vi "Download.vi"(5 "ICommunicate":refnum<class "ICommunicate.lvclass">, 7 "Node-ID":u8, 8 "error in":errorcluster, 9 "Value":variant, 10 "Multiplexer":cluster{"Index":u16, "Sub-Index":u8} {"Index" format="%.0x"}, 11 "SDO Manager in":refnum<class "SDO Manager.lvclass">) -> (0 "error out":errorcluster, 2 "Success?":bool, 3 "SDO Manager out":refnum<class "SDO Manager.lvclass">)   [LabVIEW 2024, in "CANopen Master.lvlib" / "SDO Manager.lvclass"]
uses:
  SDO Manager.lvclass
  SDO Manager.lvclass/SDO Manager.ctl
  CANopen Request/CANopen Request Message.lvclass
  Service Data Object/Service Data Object.lvclass
  CANopen Message/CANopen Message.lvclass
  HAL/Source/Interfaces/ICommunicate/ICommunicate.lvclass
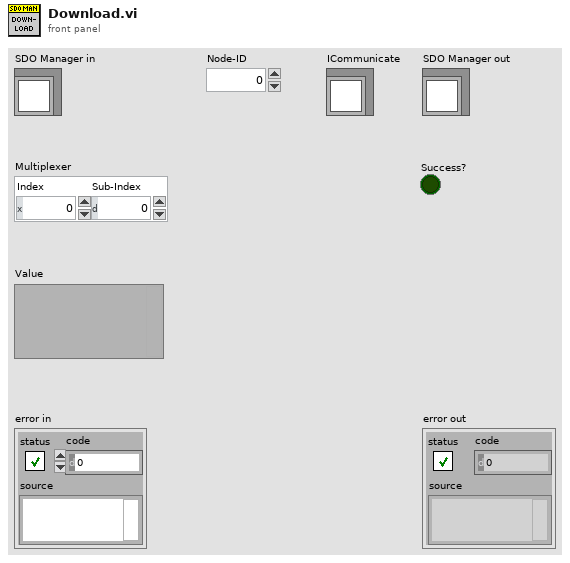
[diagram p1: front panel]
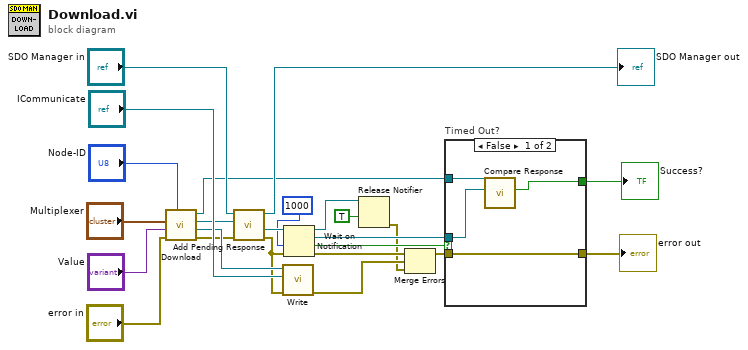
[diagram p0: block diagram]
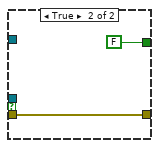
[diagram p2: hidden frame]
diagram:
  n1 = call "Download.vi"("Node-ID"="Node-ID", "error in"="error in", "Value"="Value", "Multiplexer"="Multiplexer") -> ("error out"=w7:errorcluster, "Request"=w17:refnum<class "CANopen Request Message.lvclass">, "Expected Response"=w16:refnum<class "CANopen Response Message.lvclass">, "Service Data Object out"=w12:refnum<class "Service Data Object.lvclass">)  [unwired: 4 in]
  n2 = call "Add Pending Response.vi"("Error In"=w7, "Expected Response"=w16, "reference in"="SDO Manager in") -> ("Error Out"=w3:errorcluster, "Response Notifier out"=w13:refnum<notifier>, "reference out"=→"SDO Manager out":refnum<class "SDO Manager.lvclass">)  [unwired: 6 in]
  n3 = call "Write.vi"("error in"=w3, "ICommunicate"="ICommunicate", "CANopen Message in"=w17) -> ("error out"=w2:errorcluster)  [unwired: 7 in, 1 out]
  n4 = Wait on Notification(notifier=w13, timeout in ms (-1)=1000, error in (no error)=w3) -> (notifier out=w6:refnum<notifier>, notification=w9:refnum<class "CANopen Response Message.lvclass">, timed out?=w8:bool, error out=w10:errorcluster)  [unwired: 1 in]
  n5 = Release Notifier(notifier=w6, force destroy? (F)=TRUE) -> (error out=w1:errorcluster)  [unwired: 1 in, 2 out]
  n6 = Merge Errors(w10, w2, w1) -> (w4:errorcluster)
  n7 = case "Timed Out?" shown="False" w8 {
    tunnel: w4 -> [w25 w30]
    tunnel: [w25 w30] -> w20
    tunnel: w9 -> [w27 _]
    tunnel: [w26 FALSE ("Equal?")] -> w19
    tunnel: w12 -> [w28 _]
    frame False {
      n8 = call "Compare Response.vi"("Actual"=w27, "Service Data Object"=w28) -> ("Equal?"=w26:bool)  [unwired: 8 in, 1 out]
    }
    frame True {
    }
  }
  "error out" <- w20
  "Success?" <- w19
